vi "Custom_Message.vi"(0 "Title":string, 5 "Message":string, 6 "OK Button":bool, 11 "Error_In":errorcluster, 13 "Path_Visible (F)":bool) -> (4 "Path_Out":path, 15 "Error_Out":errorcluster)   [LabVIEW 2023]
doc: "Its a custom message popup vi to prompt the user."
panel:
  in  "Path_In":path
  out "Messag_Out":string
  out "Title_Out":string
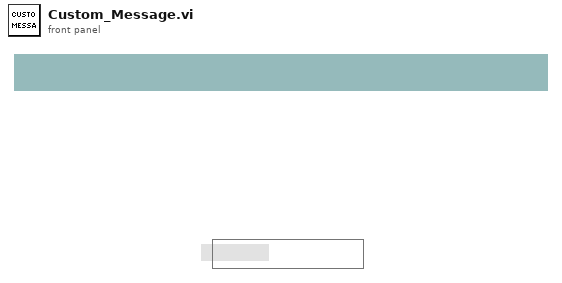
[diagram p1: front panel]
types:
  T1 = enum32{"Invalid", "Standard", "Closed", "Hidden", "Minimized", "Maximized"}
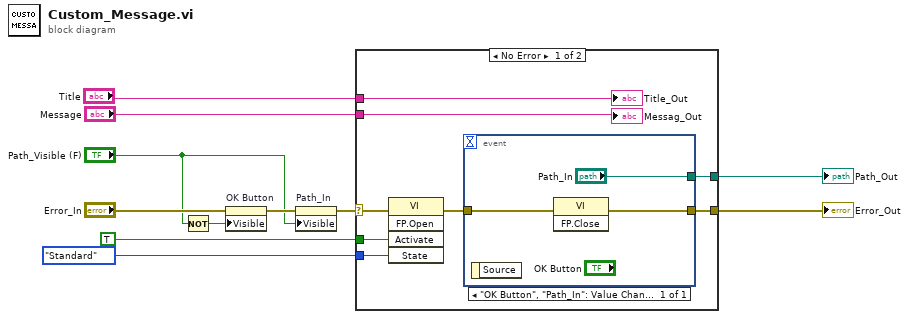
[diagram p0: block diagram]
diagram:
  n1 = Not(x="Path_Visible (F)") -> (.not. x?=w6:bool)
  n2 = property on="OK Button" class="Bool (strict)"(error in="Error_In", "Visible"=w6) -> (error out=w9:errorcluster)  [unwired: 1 in, 1 out]
  n3 = property on="Path_In" class="Path"(error in=w9, "Visible"="Path_Visible (F)") -> (error out=w7:errorcluster)  [unwired: 1 in, 1 out]
  n4 = case shown="No Error" w7 {
    selector: w7 -> [w19 w23]
    tunnel: [w15 w23] -> w3
    tunnel: TRUE ("Activate?") -> [w18 _]
    tunnel: T1."Standard" ("State") -> [w17 _]
    tunnel: [w16 _] -> w5
    tunnel: "Title" -> [w13 _]
    tunnel: "Message" -> [w12 _]
    frame No Error {
      n5 = invoke class="VI" method="FP.Open"(error in=w19, "Activate"=w18, "State"=w17) -> (error out=w14:errorcluster)  [unwired: 2 in, 4 out]
      n6 = event shown="[0] \"OK Button\", \"Path_In\": Value Change" {
        selector: _ -> [_]
        dyn-events: _ -> [_]
        timeout: _ -> [_]
        tunnel: [w22] -> w15
        tunnel: ["Path_In"] -> w16
        tunnel: w14 -> [w20]
        event "OK Button", "Path_In": Value Change {
          n7 = event-data() -> ()  [unwired: 1 in, 1 out]
          n8 = invoke class="VI" method="FP.Close"(error in=w20) -> (error out=w22:errorcluster)  [unwired: 2 in, 2 out]
        }
      }
      "Title_Out" <- w13
      "Messag_Out" <- w12
    }
    frame Error {
    }
  }
  "Error_Out" <- w3
  "Path_Out" <- w5
